vi "UnlinkNode.vi"(8 "error in":errorcluster, 10 "child in":T1, 11 "parent in":T1) -> (0 "error out":errorcluster, 2 "child out":T1, 3 "parent out":T1)   [LabVIEW 2013, in "NISE_CEF_Node.lvclass"]
doc: "Breaks the link between a child and a parent node. Removing the reference to each other in both nodes."
uses:
  NISE_CEF_Node.lvclass
  NodeRef.ctl
  NISE_CEF_Node.lvclass/NISE_CEF_Node.ctl
  ReadChildren.vi
  WriteParent.vi
  WriteChildren.vi
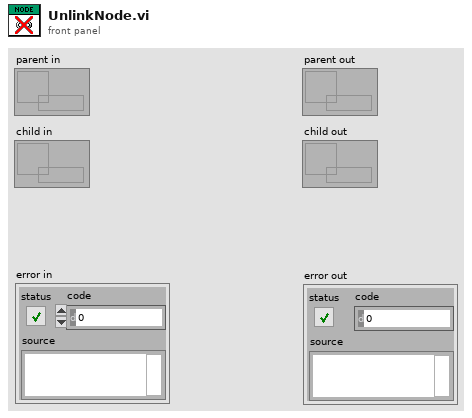
[diagram p1: front panel]
types:
  T1 = typedef "NISE_CEF_Node.lvclass/NodeRef.ctl" = refnum<data-value>
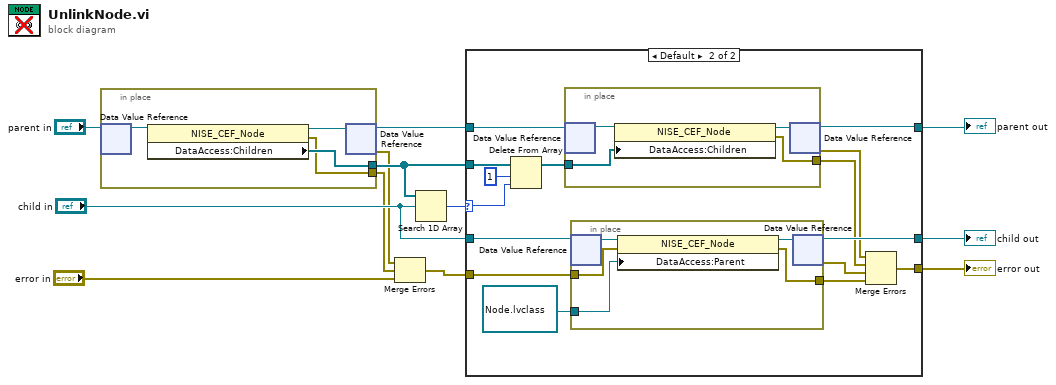
[diagram p0: block diagram]
diagram:
  n1 = in-place {
    in-place-border: [w14] -> w10
    in-place-border: [w13] -> w2
    n2 = in-place-dvr #1("parent in") -> (w16:refnum<class "NISE_CEF_Node.lvclass">)  [unwired: 1 out]
    n3 = property class="NISE_CEF_Node"(reference=w16) -> (reference out=w15:refnum<class "NISE_CEF_Node.lvclass">, error out=w13:errorcluster, "DataAccess:Children"=w14:T1[])  [unwired: 1 in]
    n4 = in-place-dvr #1(w15) -> (w11:T1, w1:errorcluster)
  }
  n5 = Merge Errors(w1, w2, "error in") -> (w3:errorcluster)
  n6 = Search 1D Array(1D array=w10, element="child in") -> (index of element=w12:i32)  [unwired: 1 in]
  n7 = case shown="Default" w12 {
    selector: w12 -> [_ w29]
    tunnel: "child in" -> [w17 w34]
    tunnel: w3 -> [w19 w33]
    tunnel: [w19 w24] -> w9
    tunnel: w11 -> [w18 w26]
    tunnel: [w18 w28] -> w5
    tunnel: [w17 w32] -> w6
    tunnel: w10 -> [_ w31]
    frame -1 {
    }
    frame Default {
      n8 = Delete From Array(array=w31, length=1, index=w29) -> (array with subset deleted=w27:T1[])  [unwired: 1 out]
      n9 = in-place {
        in-place-border: w27 -> [w36]
        in-place-border: [w35] -> w23
        n10 = in-place-dvr #2(w26) -> (w38:refnum<class "NISE_CEF_Node.lvclass">)  [unwired: 1 out]
        n11 = property class="NISE_CEF_Node"(reference=w38, "DataAccess:Children"=w36) -> (reference out=w37:refnum<class "NISE_CEF_Node.lvclass">, error out=w35:errorcluster)  [unwired: 1 in]
        n12 = in-place-dvr #2(w37) -> (w28:T1, w22:errorcluster)
      }
      n13 = in-place {
        in-place-border: w33 -> [w42]
        in-place-border: refnum<data-value> refnum ("parent out") -> [w40]
        in-place-border: [w39] -> w21
        n14 = in-place-dvr #3(w34) -> (w43:refnum<class "NISE_CEF_Node.lvclass">)  [unwired: 1 out]
        n15 = property class="NISE_CEF_Node"(reference=w43, error in=w42, "DataAccess:Parent"=w40) -> (reference out=w41:refnum<class "NISE_CEF_Node.lvclass">, error out=w39:errorcluster)
        n16 = in-place-dvr #3(w41) -> (w32:T1, w20:errorcluster)
      }
      n17 = Merge Errors(w22, w23, w20, w21) -> (w24:errorcluster)
    }
  }
  "child out" <- w6
  "parent out" <- w5
  "error out" <- w9
